vi "SimilarArraySizeFromHeader.vi"(7 "Array Element Data":variant, 8 "error in (no error)":errorcluster, 10 "Headers":string[](array[string]), 11 "Prefix Name":string) -> (0 "error out":errorcluster, 2 "1D Array of Variants Initialized":variant[](array[variant]))   [LabVIEW 2014, in "TableLogger_Actor.lvlib" / "TableLogger_Actor.lvclass"]
uses:
  TableLogger_Actor.lvclass
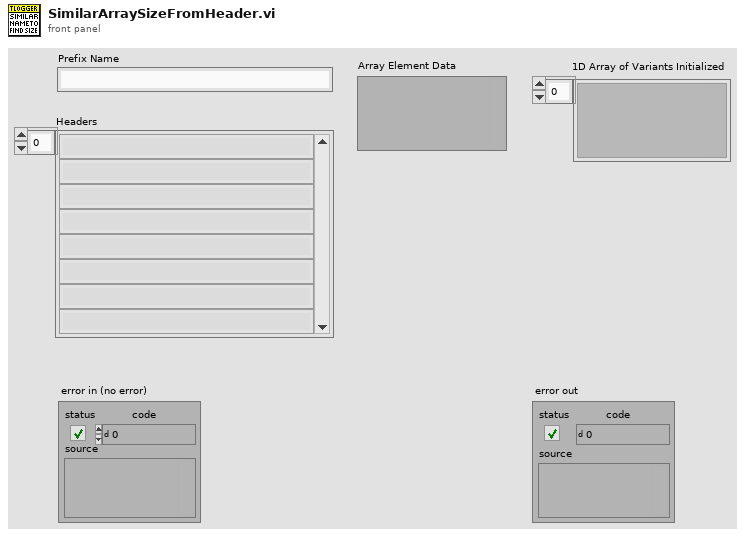
[diagram p1: front panel]
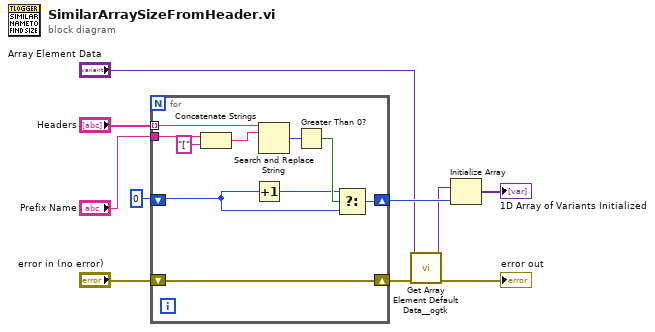
[diagram p0: block diagram]
diagram:
  n1 = for {
    tunnel: "Headers" -> [w14] mode=indexing
    tunnel: "Prefix Name" -> [w20]
    shift-right: [w17] -> w6
    shift-left: 0 ("index") -> [w16]
    shift-right: [w11] -> w2
    shift-left: "error in (no error)" -> [w11]
    n2 = Concatenate Strings(w20, "[" ("string")) -> (w13:string)
    n3 = Increment(x=w16) -> (x+1=w15:i32)
    n4 = Search and Replace String(input string=w14, search string=w13) -> (number of replacements=w19:i32)  [unwired: 6 in, 3 out]
    n5 = Greater Than 0?(x=w19) -> (x > 0?=w18:bool)
    n6 = Select(t=w15, s=w18, f=w16) -> (s? t:f=w17:i32)
  }
  n7 = call <userlib>:"Get Array Element Default Data__ogtk.vi"("error in (no error)"=w2, "Array"="Array Element Data") -> ("error out"=→"error out":errorcluster, "Array Element Default Data"=w3:variant)  [unwired: 8 in]
  n8 = Initialize Array(w3, w6) -> (→"1D Array of Variants Initialized":variant[])
